vi "Test Basic operations 1.vi"() -> ()   [LabVIEW 2014]
uses:
  <vilib>/Aledyne-TSXperts/Arduino Compatible Compiler for LabVIEW/addons/Complex Numbers/Complex Numbers.lvlib
panel:
  out "tanh(A)":u32
  out "csch(A)":u32
  out "reciprocal A":u32
  out "cotan(A)":u32
  out "arcsinh(A)":u32
  out "Error Out":errorcluster
  in  "error in (no error)":errorcluster
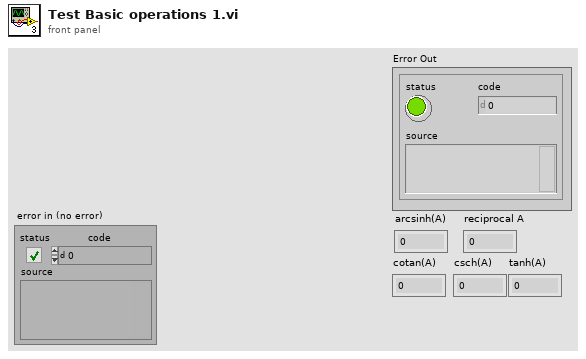
[diagram p1: front panel]
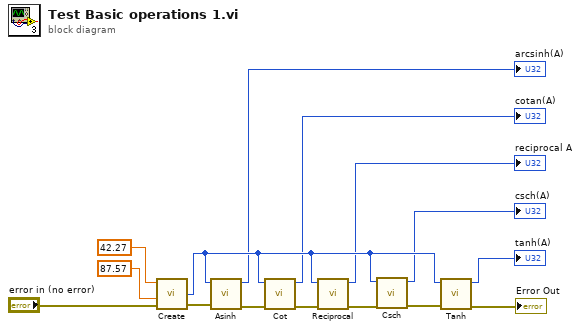
[diagram p0: block diagram]
diagram:
  n1 = call <vilib>:"Create.vi"("Error In"="error in (no error)", "Imag"=87.57, "Real"=42.27) -> ("Error Out"=w12:errorcluster, "Complex"=w7:u32)  [unwired: 2 in]
  n2 = call <vilib>:"Asinh.vi"("Error In"=w12, "A"=w7) -> ("Error Out"=w11:errorcluster, "arcsinh(A)"=→"arcsinh(A)":u32)  [unwired: 8 in]
  n3 = call <vilib>:"Cot.vi"("Error In"=w11, "A"=w7) -> ("Error Out"=w10:errorcluster, "cotan(A)"=→"cotan(A)":u32)  [unwired: 8 in]
  n4 = call <vilib>:"Reciprocal.vi"("Error In"=w10, "A"=w7) -> ("Error Out"=w9:errorcluster, "reciprocal A"=→"reciprocal A":u32)  [unwired: 8 in]
  n5 = call <vilib>:"Csch.vi"("Error In"=w9, "A"=w7) -> ("Error Out"=w8:errorcluster, "csch(A)"=→"csch(A)":u32)  [unwired: 8 in]
  n6 = call <vilib>:"Tanh.vi"("Error In"=w8, "A"=w7) -> ("Error Out"=→"Error Out":errorcluster, "tanh(A)"=→"tanh(A)":u32)  [unwired: 8 in]
